vi "GSI-HVSwitch2.reset.vi"(0 "i ref in":refnum<vi>, 3 "ms timeout (10000)":i32=10000, 5 "error in (no error)":errorcluster) -> (14 "i ref out":refnum<vi>, 17 "timed out":bool, 19 "error out":errorcluster)   [LabVIEW 2014, in "GSI-HVSwitch2.lvlib"]
doc: "Resets a GSI-HVSwitch2 by performing an \"emergency off\"."
uses:
  GSI-HVSwitch2.lvlib
  GSI-HVSwitch2.mode.ctl
  CSinstr.lib/SDEX/SDEX.revisionType.ctl
  CSCore/CSApplicationBaseClasses/PSChannelBase/PSChannelBase.statusType.ctl
  CSCore/CSApplicationBaseClasses/PSChannelBase/PSChannelBase.directionType.ctl
  CSCore/CSApplicationBaseClasses/PSChannelBase/PSChannelBase.serviceType.ctl
  CSCore/CSApplicationBaseClasses/DeviceBase/DeviceBase.lvlib
  CSCore/CSApplicationBaseClasses/PSChannelBase/PSChannelBase.lvlib
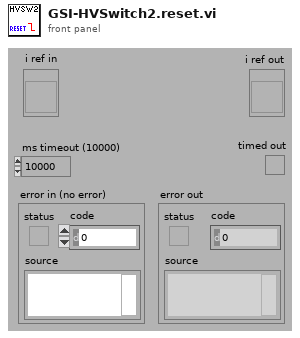
[diagram p1: front panel]
types:
  T1 = typedef "SDEXDriver.lvlib/SDEX.revisionType.ctl" = enum16{"unknown", "hvamp3", "hvswi1", "htrp0", "WDG0"}
  T2 = typedef "GSI-HVSwitch2.lvlib/GSI-HVSwitch2.mode.ctl" = enum16{"unknown", "switch", "stepper"}
  T3 = typedef "PSChannelBase.lvlib/PSChannelBase.serviceType.ctl" = enum16{"onOff", "voltage", "current", "tripCurrent", "rampUpSpeed", "rampDownSpeed", "status"}
  T4 = typedef "GSI-HVSwitch2.lvlib/GSI-HVSwitch2.i attribute.ctl" = cluster{"SDEX VISA Cluster":T5, "SetVoltage SW0":dbl, "SetVoltage SW1":dbl, "ActTempAmp":dbl, "ActTempPS1":dbl, "ActTempPS2":dbl, "mode":T2, "interfaceInitialized":bool, "serviceIDs":cluster{"nomVoltage0ID":i32, "nomVoltage1ID":i32, "actTempAmpID":i32, "actTempPS1ID":i32, "actTempPS2ID":i32, "modeID":i32}, "usedChannels":i32}
  T5 = typedef "SDEXDriver.lvlib/SDEX.VISA Control.ctl" = cluster{"VISA resource name":refnum<visa-resource-name>, "HEX address":u16, "VISA Timeout Value (1000 ms)":u32, "Lock Timeout (1000 ms)":u32, "semaphore":T6, "Baud rate":u32, "revision":T1, "deviceInfo":string}
  T6 = typedef "Semaphore RefNum" = refnum<k1>
  T7 = typedef "PSChannelBase.lvlib/PSChannelBase.directionType.ctl" = enum16{"unknown", "update actual value", "update nominal value", "update both"}
  T8 = typedef "PSChannelBase.lvlib/PSChannelBase.statusType.ctl" = i32
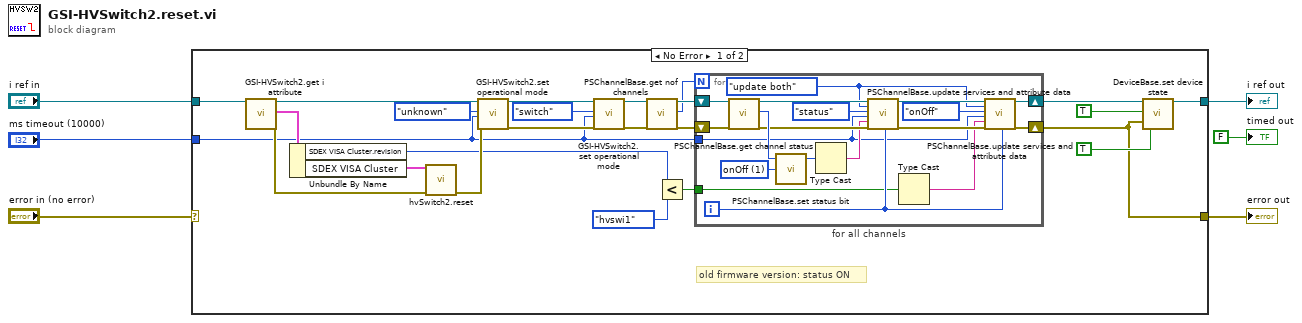
[diagram p0: block diagram]
diagram:
  n1 = case shown="No Error" "error in (no error)" {
    selector: "error in (no error)" -> [_ w50]
    tunnel: "i ref in" -> [w27 w51]
    tunnel: [w30 w51] -> w5
    tunnel: "ms timeout (10000)" -> [w12 _]
    tunnel: [w7 w50] -> w2
    frame No Error {
      # "old firmware version: status ON"
      n2 = call "GSI-HVSwitch2.get i attribute.vi"("i ref in"=w27) -> ("i ref out"=w22:refnum<vi>, "i attribute"=w26:T4, "error out"=w24:errorcluster)  [unwired: 16 in]
      n3 = Unbundle By Name(w26) -> ("SDEX VISA Cluster.revision"=w11:T1, "SDEX VISA Cluster"=w25:T5)
      n4 = call "hvSwitch2.reset.vi"("SDEX VISA Cluster"=w25, "error in (no error)"=w24) -> ("error out"=w21:errorcluster)  [unwired: 12 in, 1 out]
      n5 = call "GSI-HVSwitch2.set operational mode.vi"("i ref in"=w22, "mode"=GSI-HVSwitch2.mode."unknown", "ms timeout (10000)"=w12, "error in (no error)"=w21) -> ("i ref out"=w18:refnum<vi>, "error out"=w19:errorcluster)  [unwired: 13 in, 1 out]
      n6 = call "GSI-HVSwitch2.set operational mode.vi"("i ref in"=w18, "mode"=GSI-HVSwitch2.mode."switch", "ms timeout (10000)"=w12, "error in (no error)"=w19) -> ("i ref out"=w16:refnum<vi>, "error out"=w17:errorcluster)  [unwired: 13 in, 1 out]
      n7 = call "PSChannelBase.get nof channels.vi"("i ref in"=w16, "error in (no error)"=w17) -> ("i ref out"=w15:refnum<vi>, "NofChannels"=w13:i32, "error out"=w14:errorcluster)  [unwired: 15 in]
      n8 = Less?(x=w11, y=SDEX.revisionType."hvswi1") -> (x < y?=w9:bool)
      n9 = for "for all channels" {
        N: w13 -> [_]
        shift-right: [w35] -> w7
        shift-left: w14 -> [w48]
        shift-right: [w36] -> w8
        shift-left: w15 -> [w49]
        tunnel: w12 -> [w38]
        tunnel: w9 -> [w32]
        i -> [w40]
        w34 = PSChannelBase.directionType."update both" ("direction")
        w46 = T8 1 items=["onOff"=1, "inRange"=2, "rampingUp"=4, "rampingDown"=8, "currentRegulated"=16, "voltageRegulated"=32, "reserved1"=64, "reserved2"=128, "reserved3"=256, "reserved4"=512, "reserved5"=1024, "reserved6"=2048, "reserved7"=4096, "reserved8"=8192, "reserved9"=16384, "reserved10"=32768, "reserved11"=65536, "user1"=131072, "user2"=262144, "user3"=524288, "user4"=1048576, "user5"=2097152, "user6"=4194304, "user7"=8388608, "user8"=16777216, "user9"=33554432, "user10"=67108864, "user11"=134217728, "tripped"=268435456, "warning"=536870912, "error"=1073741824] ("statusBit")
        n10 = call "PSChannelBase.get channel status.vi"("i ref in"=w49, "error in (no error)"=w48) -> ("i ref out"=w45:refnum<vi>, "status"=w47:i32, "error out"=w44:errorcluster)  [unwired: 15 in]
        n11 = call "PSChannelBase.set status bit.vi"("statusBit"=w46, "status"=w47) -> ("status out"=w42:T8)  [unwired: 3 in]
        n12 = Type Cast(x=w42) -> (*(type *) &x=w41:string)  [unwired: 1 in]
        n13 = call "PSChannelBase.update services and attribute data.vi"("i ref in"=w45, "direction"=w34, "service"=PSChannelBase.serviceType."status", "ms timeout (10000)"=w38, "value"=w41, "error in (no error)"=w44, "channelNumber"=w40) -> ("i ref out"=w37:refnum<vi>, "error out"=w39:errorcluster)  [unwired: 10 in, 1 out]
        n14 = Type Cast(x=w32) -> (*(type *) &x=w31:string)  [unwired: 1 in]
        n15 = call "PSChannelBase.update services and attribute data.vi"("i ref in"=w37, "direction"=w34, "service"=PSChannelBase.serviceType."onOff", "ms timeout (10000)"=w38, "value"=w31, "error in (no error)"=w39, "channelNumber"=w40) -> ("i ref out"=w36:refnum<vi>, "error out"=w35:errorcluster)  [unwired: 10 in, 1 out]
      }
      n16 = call "DeviceBase.set device state.vi"("i ref in"=w8, "implicit"=TRUE, "device error"=w7, "mayResetError (FALSE)"=TRUE) -> ("i ref out"=w30:refnum<vi>)  [unwired: 13 in, 2 out]
    }
    frame Error {
    }
  }
  "error out" <- w2
  "i ref out" <- w5
  "timed out" <- FALSE ("timed out")
